vi "Tloop.vi"(0 "ITCSignal":T1={"ITC"=0, "Signal"=enum."Sensor 3"}, 1 "T target [K]":dbl=1.8, 2 "Precision":dbl=0.2, 3 "Time limit":dbl=3600.0, 4 "Regulate ?":bool) -> (5 "ITCSignal 2":T1={"ITC"=0, "Signal"=enum."Sensor 1"}, 6 "Finish":bool)   [LabVIEW 2011]
uses:
  Kelvinox drivers/ITCAPPS - Copie.LLB/ITCSignal.ctl
  Kelvinox drivers/ITCAPPS.LLB/ITCSignals.ctl
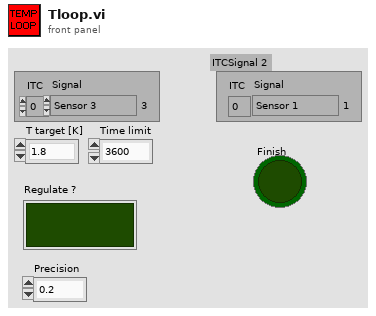
[diagram p1: front panel]
types:
  T1 = typedef "ITCSignal.ctl" = cluster{"ITC":u16, "Signal":T2}
  T2 = typedef "ITCSignals.ctl" = enum16{"Setpoint", "Sensor 1", "Sensor 2", "Sensor 3", "Needle Valve %", "Heater %"}
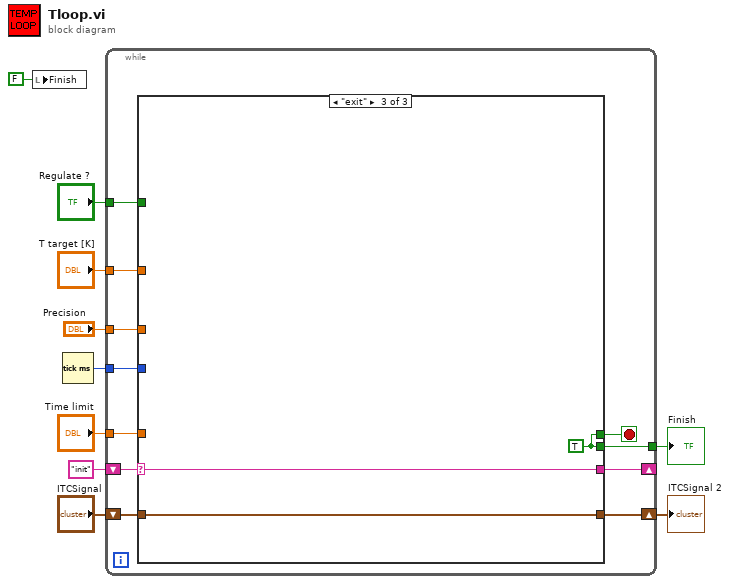
[diagram p0: block diagram]
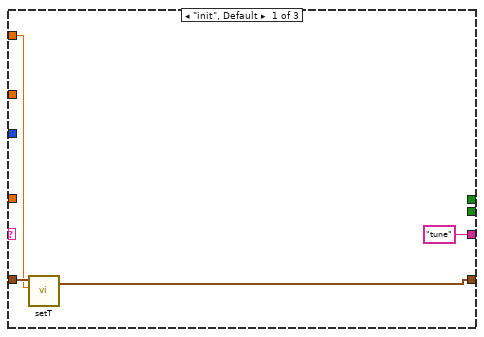
[diagram p2: hidden frame]
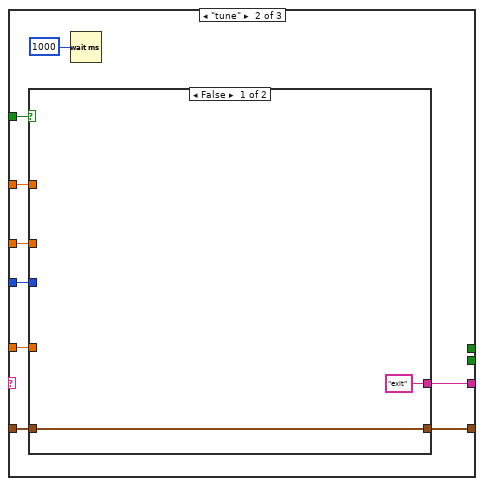
[diagram p3: hidden frame]
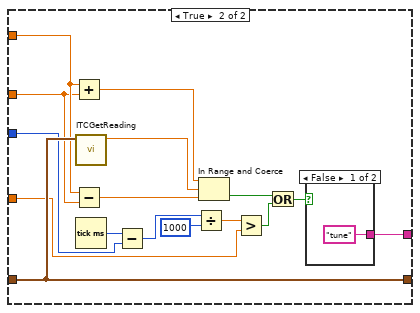
[diagram p4: hidden frame]
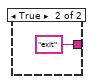
[diagram p5: hidden frame]
diagram:
  n1 = local write "Finish"(FALSE ("Finish")) -> ()
  n2 = Tick Count (ms)() -> (millisecond timer value=w4:u32)
  n3 = while {
    shift-right: [w17] -> _
    shift-left: "init" -> [w21]
    tunnel: "T target [K]" -> [w19]
    shift-right: [w18] -> w6
    shift-left: "ITCSignal" -> [w20]
    tunnel: "Regulate ?" -> [w16]
    tunnel: "Precision" -> [w14]
    tunnel: w4 -> [w13]
    tunnel: "Time limit" -> [w12]
    tunnel: [w11] -> w2
    stop <- w15 stop-if-true
    n4 = case shown="\"exit\"" w21 {
      selector: w21 -> [_ _ w57]
      tunnel: w20 -> [w25 w32 w55]
      tunnel: w19 -> [w24 w30 _]
      tunnel: [w23 w31 w55] -> w18
      tunnel: ["tune" w33 w57] -> w17
      tunnel: w16 -> [_ w34 _]
      tunnel: [_ _ w56] -> w15
      tunnel: w14 -> [_ w29 _]
      tunnel: w13 -> [_ w27 _]
      tunnel: w12 -> [_ w26 _]
      tunnel: [_ _ w56] -> w11
      frame "init", Default {
        n5 = call "setT.vi"("ITCSignal"=w25, "T target [K]"=w24) -> ("ITCSignal 2"=w23:T1)  [unwired: 3 in, 1 out]
      }
      frame "tune" {
        n6 = case shown="False" w34 {
          tunnel: ["exit" w46] -> w33
          tunnel: w32 -> [w35 w52]
          tunnel: [w35 w52] -> w31
          tunnel: w30 -> [_ w50]
          tunnel: w29 -> [_ w49]
          tunnel: w27 -> [_ w44]
          tunnel: w26 -> [_ w37]
          frame False {
          }
          frame True {
            n7 = Add(x=w50, y=w49) -> (x+y=w47:dbl)
            n8 = Subtract(x=w50, y=w49) -> (x-y=w48:dbl)
            n9 = call "ITCGetReading.vi"("Signal"=w52) -> ("Reading"=w51:dbl)  [unwired: 6 in]
            n10 = Tick Count (ms)() -> (millisecond timer value=w45:u32)
            n11 = Subtract(x=w45, y=w44) -> (x-y=w43:u32)
            n12 = Divide(x=w43, y=u32 1000) -> (x/y=w39:dbl)
            n13 = In Range and Coerce(upper limit=w47, x=w51, lower limit=w48) -> (In Range?=w41:bool)  [unwired: 1 out]
            n14 = Greater?(x=w39, y=w37) -> (0:w38:bool)
            n15 = Or(x=w41, y=w38) -> (x .or. y?=w40:bool)
            n16 = case shown="False" w40 {
              tunnel: ["tune" "exit"] -> w46
              frame False {
              }
              frame True {
              }
            }
          }
        }
        n17 = Wait (ms)(milliseconds to wait=u32 1000) -> ()  [unwired: 1 out]
      }
      frame "exit" {
        w56 = TRUE
      }
    }
  }
  "ITCSignal 2" <- w6
  "Finish" <- w2
